vi "Retrieve File Change Info.vi"(8 "error in (no error)":errorcluster {"code" format="Error %.0f"}, 10 "Absolute File Path":path, 11 "VIDoc Printer - Confluence In":refnum<class "VIDoc Printer - Confluence.lvclass">) -> (0 "error out":errorcluster {"code" format="Error %.0f"}, 1 "File Change Info Available?":bool, 2 "File Change Info":T1, 3 "VIDoc Printer - Confluence Out":refnum<class "VIDoc Printer - Confluence.lvclass">)   [LabVIEW 2023, in "VIDoc Printer - Confluence.lvlib" / "VIDoc Printer - Confluence.lvclass"]
uses:
  VIDoc Printer - Confluence.lvclass
  VIDoc Printer - Confluence.lvclass/VIDoc Printer - Confluence.ctl
  Accessors/Get File Change Map.vi
  Accessors/Get Working Directory.vi
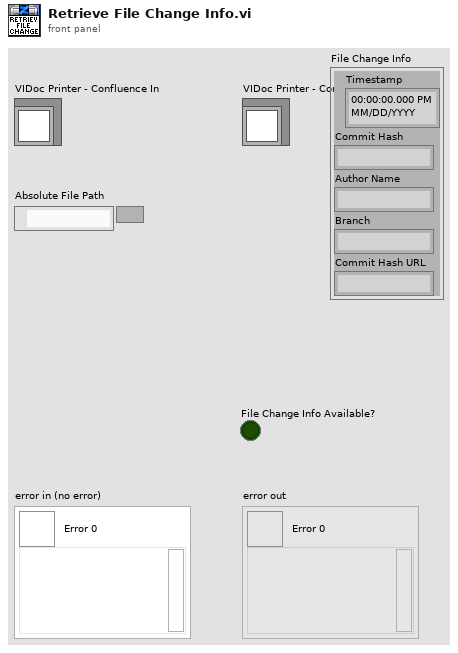
[diagram p1: front panel]
types:
  T1 = cluster{"Timestamp":timestamp, "Commit Hash":string, "Author Name":string, "Branch":string, "Commit Hash URL":string}
  T2 = typedef "File Change Map.ctl" = map{string, cluster{"Timestamp":timestamp, "Commit Hash":string, "Author Name":string, "Branch":string, "Commit Hash URL":string}}
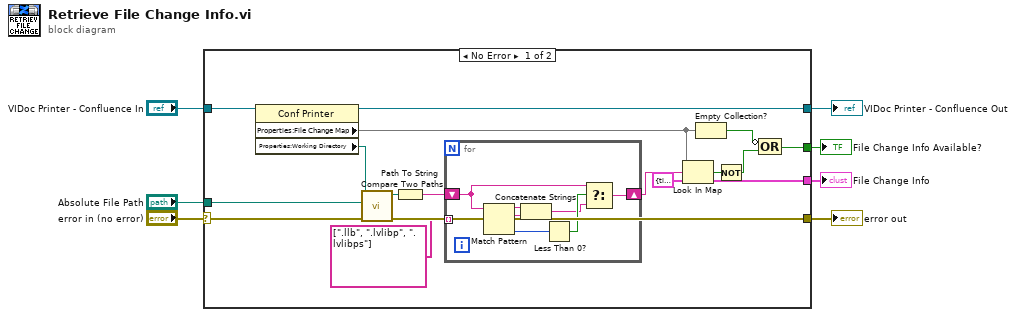
[diagram p0: block diagram]
diagram:
  n1 = case shown="No Error" "error in (no error)" {
    selector: "error in (no error)" -> [w22 w34]
    tunnel: [w21 w34] -> w6
    tunnel: [w23 w33] -> w4
    tunnel: "VIDoc Printer - Confluence In" -> [w24 w33]
    tunnel: "Absolute File Path" -> [w19 _]
    tunnel: [w17 _] -> w1
    tunnel: [w12 _] -> w2
    frame No Error {
      n2 = property class="Conf Printer"(reference=w24) -> (reference out=w23:refnum<class "VIDoc Printer - Confluence.lvclass">, "Properties:File Change Map"=w14:T2, "Properties:Working Directory"=w20:path)  [unwired: 1 in, 1 out]
      n3 = call <vilib>:"Compare Two Paths.vi"("error in (no error)"=w22, "Path 2"=w19, "Path 1"=w20) -> ("error out"=w21:errorcluster, "Relative Path from 1 to 2"=w18:path)  [unwired: 5 in, 2 out]
      n4 = Path To String(path=w18) -> (string=w10:string)
      n5 = for {
        shift-right: [w32] -> w8
        shift-left: w10 -> [w31]
        tunnel: string[] [".llb", ".lvlibp", ".lvlibps"] ("regular expression") -> [w30] mode=indexing
        n6 = Match Pattern(string=w31, regular expression=w30) -> (before substring=w27:string, match substring=w26:string, offset past match=w29:i32)  [unwired: 1 in, 1 out]
        n7 = Concatenate Strings(w27, w26) -> (w25:string)
        n8 = Less Than 0?(x=w29) -> (x < 0?=w28:bool)
        n9 = Select(t=w31, s=w28, f=w25) -> (s? t:f=w32:string)
      }
      n10 = Look In Map(map=w14, key=w8, default value=T1 {"Timestamp"=timestamp(0 s since 1904-01-01), "Commit Hash"="N/A", "Author Name"="N/A", "Branch"="Uncommitted", "Commit Hash URL"=""}) -> (key not found?=w16:bool, value=w17:T1)
      n11 = Empty Collection?(1:w14) -> (0:w11:bool)
      n12 = Not(x=w16) -> (.not. x?=w15:bool)
      n13 = Compound Arithmetic op=OR(invert w11, w15) -> (w12:bool)
    }
    frame Error {
    }
  }
  "error out" <- w6
  "VIDoc Printer - Confluence Out" <- w4
  "File Change Info Available?" <- w2
  "File Change Info" <- w1
